vi "53230A_Freq_Measure.vi"(0 "VISA resource name":refnum<visa-resource-name>, 5 "Timeout (10000 ms)":u32=10000, 11 "error in (no error)":errorcluster) -> (3 "Minimum":dbl format="%#_12g", 4 "VISA resource name out":refnum<visa-resource-name>, 6 "Mean":dbl format="%#_12g", 8 "status":bool, 10 "Standard Deviation":dbl, 13 "Allan_Dev":dbl format="%#_12g", 14 "Maximum":dbl format="%#_12g", 15 "error out":errorcluster)   [LabVIEW 2016]
doc: "Performs a single, new measurement and outputs measurement statistics."
uses:
  <userlib>/_TI-LA/Instr Drivers/Counter/E532XX/Driver/Base/Public/Data/Low Level/Fetch Measurement (Statistics).vi
  <userlib>/_TI-LA/Instr Drivers/Counter/E532XX/Driver/Base/Agilent 532XX Series.lvlib
panel:
  out "Execution Time":u32
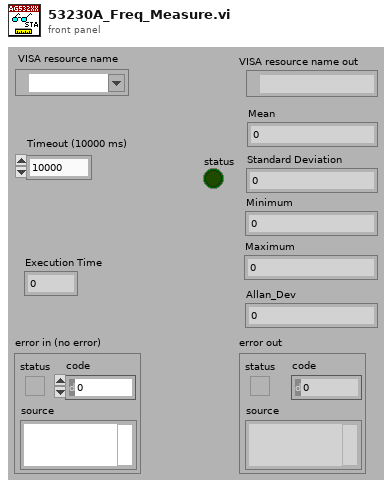
[diagram p1: front panel]
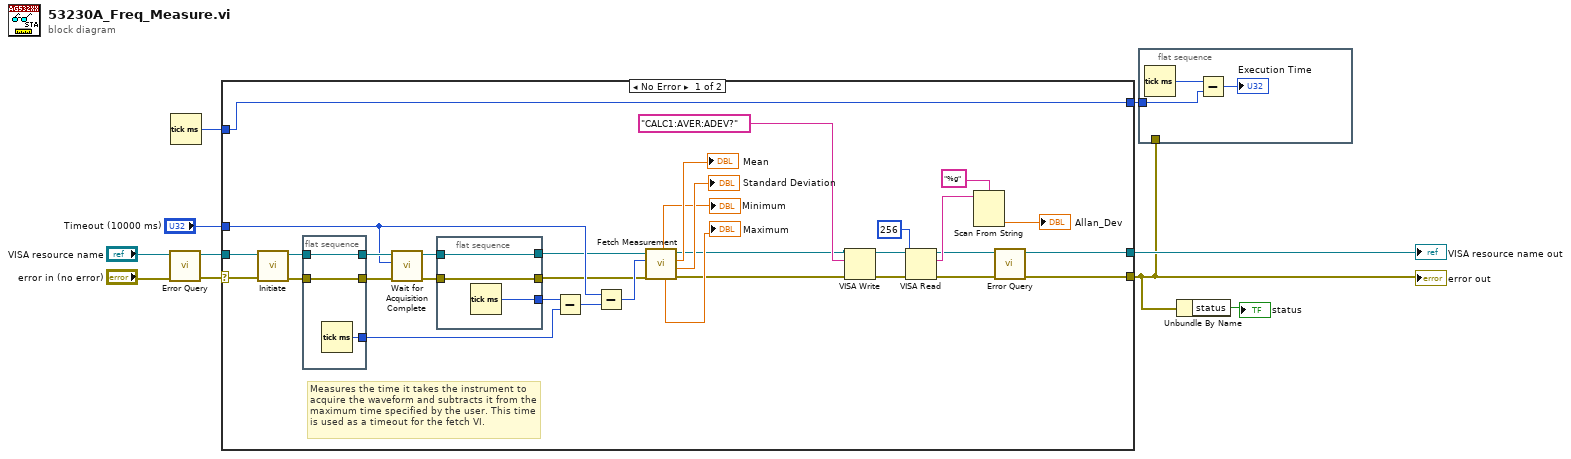
[diagram p0: block diagram]
diagram:
  n1 = call <userlib>:"Error Query.vi"("error in (no error)"="error in (no error)", "VISA resource name"="VISA resource name") -> ("error out"=w4:errorcluster, "VISA resource name out"=w6:refnum<visa-resource-name>)  [unwired: 8 out]
  n2 = Tick Count (ms)() -> (millisecond timer value=w3:u32)
  n3 = case shown="No Error" w4 {
    selector: w4 -> [w12 w52]
    tunnel: [w43 w51] -> w10
    tunnel: "Timeout (10000 ms)" -> [w36 _]
    tunnel: [w25 w52] -> w1
    tunnel: w6 -> [w13 w51]
    tunnel: w3 -> [w11 w50]
    tunnel: [w11 w50] -> w2
    frame No Error {
      # "Measures the time it takes the instrument to acquire the waveform and subtracts it from the maximum time specified by the user. This time is used as a timeout for the fetch VI."
      n4 = call <userlib>:"Initiate.vi"("error in (no error)"=w12, "VISA resource name"=w13) -> ("error out"=w40:errorcluster, "VISA resource name out"=w41:refnum<visa-resource-name>)  [unwired: 8 out]
      n5 = flat-sequence {
        tunnel: [w49] -> w37
        tunnel: w41 -> [w49]
        tunnel: [w48] -> w38
        tunnel: w40 -> [w48]
        tunnel: [w47] -> w39
        frame #0 {
          n6 = Tick Count (ms)() -> (millisecond timer value=w47:u32)
        }
      }
      n7 = call <userlib>:"Wait for Acquisition Complete.vi"("error in (no error)"=w38, "Maximum Time (10000 ms)"=w36, "VISA resource name"=w37) -> ("error out"=w34:errorcluster, "VISA resource name out"=w35:refnum<visa-resource-name>)  [unwired: 1 in, 6 out]
      n8 = flat-sequence {
        tunnel: [w46] -> w30
        tunnel: w35 -> [w46]
        tunnel: [w45] -> w31
        tunnel: w34 -> [w45]
        tunnel: [w44] -> w33
        frame #0 {
          n9 = Tick Count (ms)() -> (millisecond timer value=w44:u32)
        }
      }
      n10 = Subtract(x=w33, y=w39) -> (x-y=w42:u32)
      n11 = Subtract(x=w36, y=w42) -> (x-y=w32:u32)
      n12 = call-poly <userlib>:"Fetch Measurement.vi"("error in (no error)"=w31, "Timeout (10000 ms)"=w32, "VISA resource name"=w30) -> ("error out"=w17:errorcluster, "Standard Deviation"=→"Standard Deviation":dbl, "Mean"=→"Mean":dbl, "VISA resource name out"=w18:refnum<visa-resource-name>, "Maximum"=→"Maximum":dbl, "Minimum"=→"Minimum":dbl)  [unwired: 3 out]
      n13 = VISA Write(VISA resource name=w18, write buffer="CALC1:AVER:ADEV?", error in (no error)=w17) -> (VISA resource name out=w23:refnum<visa-resource-name>, error out=w22:errorcluster)  [unwired: 1 out]
      n14 = VISA Read(VISA resource name=w23, byte count=u32 256, error in (no error)=w22) -> (VISA resource name out=w15:refnum<visa-resource-name>, read buffer=w20:string, error out=w16:errorcluster)  [unwired: 1 out]
      n15 = Scan From String(format string="%g", input string=w20) -> (output 1=→"Allan_Dev":dbl)  [unwired: 3 in, 3 out]
      n16 = call <userlib>:"Error Query.vi"("error in (no error)"=w16, "VISA resource name"=w15) -> ("error out"=w25:errorcluster, "VISA resource name out"=w43:refnum<visa-resource-name>)  [unwired: 8 out]
    }
    frame Error {
    }
  }
  "error out" <- w1
  "VISA resource name out" <- w10
  n17 = flat-sequence {
    tunnel: w2 -> [w55]
    tunnel: [w53] -> _
    tunnel: w1 -> [w53]
    frame #0 {
      n18 = Tick Count (ms)() -> (millisecond timer value=w56:u32)
      n19 = Subtract(x=w56, y=w55) -> (x-y=→"Execution Time":u32)
    }
  }
  n20 = Unbundle By Name(w1) -> ("status"=→"status":bool)
